vi "locate engine.vi"(8 "error in":errorcluster, 11 "component":T1) -> (0 "error out":errorcluster, 3 "engine":refnum<data-value>)   [LabVIEW 2013, in "PL Framework Configuration Tool.lvlib" / "module editor node.lvclass"]
uses:
  module editor node.lvclass
  Engine Parent/Engine Parent Editor Node.lvclass
  <vilib>/NI/Configuration Framework/Node/NodeRef.ctl
  <vilib>/NI/Configuration Framework/Node/NISE_CEF_Node.lvclass
  <vilib>/NI/Configuration Framework/Node/NISE_CEF_Node.lvclass/NISE_CEF_Node.ctl
  <vilib>/NI/Configuration Framework/Node/ReadParent.vi
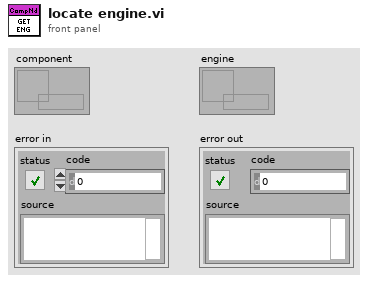
[diagram p1: front panel]
types:
  T1 = typedef "NISE_CEF_Node.lvclass/NodeRef.ctl" = refnum<data-value>
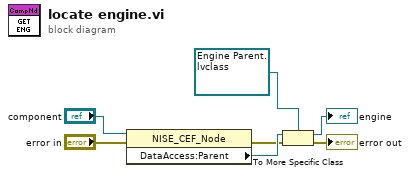
[diagram p0: block diagram]
diagram:
  n1 = property class="NISE_CEF_Node"(reference="component", error in="error in") -> (error out=w4:errorcluster, "DataAccess:Parent"=w5:T1)  [unwired: 1 out]
  n2 = To More Specific Class(target class=refnum<data-value> refnum ("data value reference"), reference=w5, error in=w4) -> (specific class reference=→"engine":refnum<data-value>, error out=→"error out":errorcluster)
